vi "Test 7.vi"() -> ()   [LabVIEW 2015, in "Drona basic.lvlib"]
uses:
  Drona basic.lvlib
panel:
  out "Label.Text 2":string
  out "Label.Text":string
  in  "Cluster":T1
  out "error out":errorcluster
  in  "error in (no error)":errorcluster
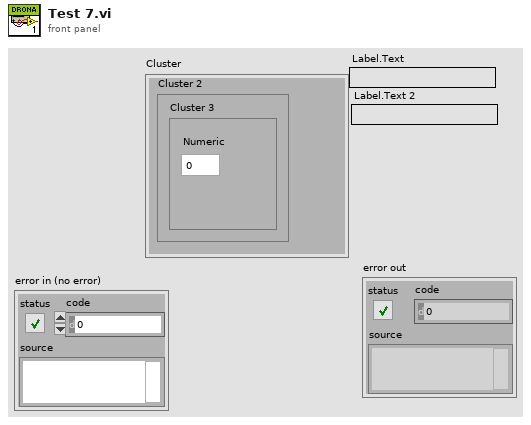
[diagram p1: front panel]
types:
  T1 = cluster{"Cluster 2":cluster{"Cluster 3":cluster{"Numeric":dbl}}}
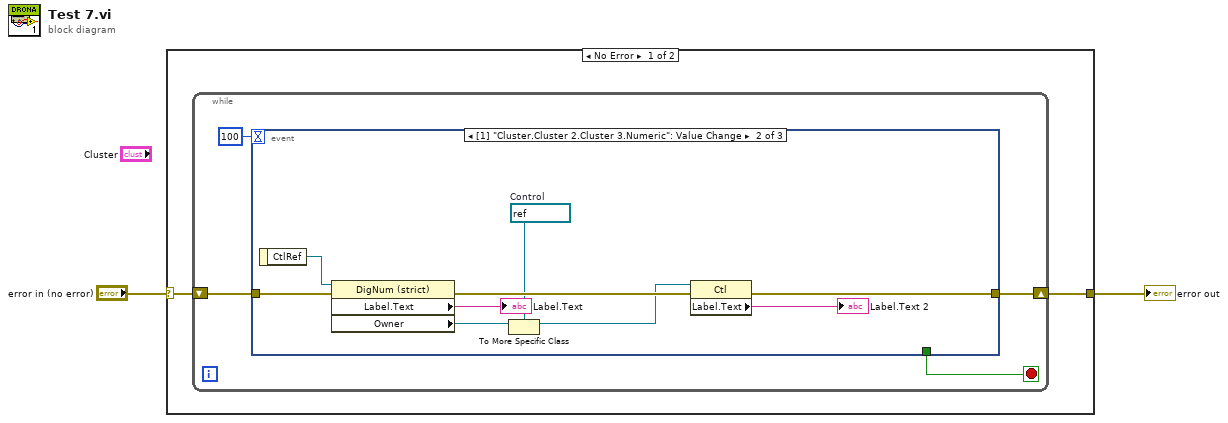
[diagram p0: block diagram]
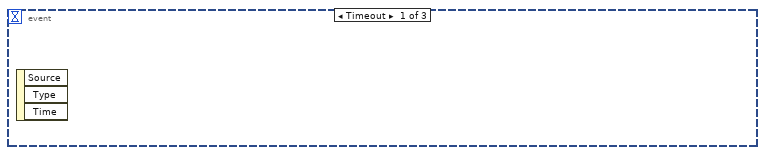
[diagram p2: hidden frame]
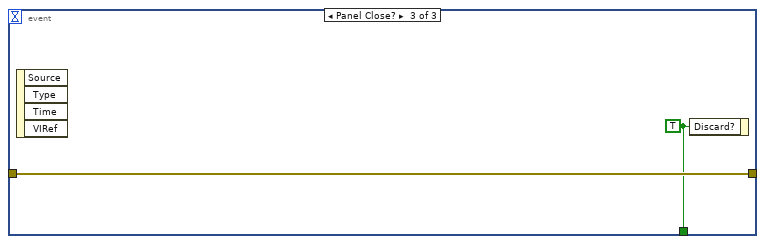
[diagram p3: hidden frame]
diagram:
  n1 = case shown="No Error" "error in (no error)" {
    selector: "error in (no error)" -> [w4 w20]
    tunnel: [w3 w20] -> w1
    frame No Error {
      n2 = while {
        shift-right: [w7] -> w3
        shift-left: w4 -> [w8]
        stop <- w5 stop-if-true
        n3 = event shown="[1] \"Cluster.Cluster 2.Cluster 3.Numeric\": Value Change" {
          selector: _ -> [_ _ _]
          dyn-events: _ -> [_ _ _]
          timeout: 100 -> [_ _ _]
          tunnel: w8 -> [_ w17 w19]
          tunnel: [_ w13 w19] -> w7
          tunnel: [_ _ w18] -> w5
          event Timeout {
            n4 = event-data() -> ()  [unwired: 1 in, 3 out]
          }
          event "Cluster.Cluster 2.Cluster 3.Numeric": Value Change {
            w9 = refnum<vi> refnum  # Control
            n5 = event-data() -> ("CtlRef"=w14:refnum<vi>)  [unwired: 1 in]
            n6 = property class="DigNum (strict)"(reference=w14, error in=w17) -> (error out=w16:errorcluster, "Label.Text"=→"Label.Text":string, "Owner"=w12:refnum<vi>)  [unwired: 1 out]
            n7 = To More Specific Class(target class=w9, reference=w12) -> (specific class reference=w10:refnum<vi>)  [unwired: 1 in, 1 out]
            n8 = property class="Ctl"(reference=w10, error in=w16) -> (error out=w13:errorcluster, "Label.Text"=→"Label.Text 2":string)  [unwired: 1 out]
          }
          event Panel Close? {
            w18 = TRUE ("Discard?")
            n9 = event-data() -> ()  [unwired: 1 in, 4 out]
            n10 = event-data("Discard?"=w18) -> ()  [unwired: 1 in, 1 out]
          }
        }
      }
    }
    frame Error {
    }
  }
  "error out" <- w1
